vi "TypeDescriptor_GetDefault.vi"(11 "type descriptor":i16[](array[numeric])) -> (0 "error out":errorcluster, 2 "Default":variant, 3 "type descriptor dup":i16[](array[numeric]))   [LabVIEW 2013, in "OpenDescriptor.lvlib"]
uses:
  OpenDescriptor.lvlib
  <vilib>/Utility/error.llb/Error Cluster From Error Code.vi
  <vilib>/ErrorRing/Error Ring.xnode
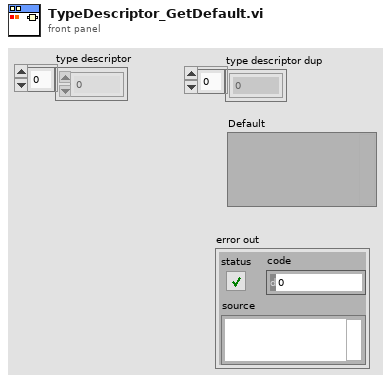
[diagram p1: front panel]
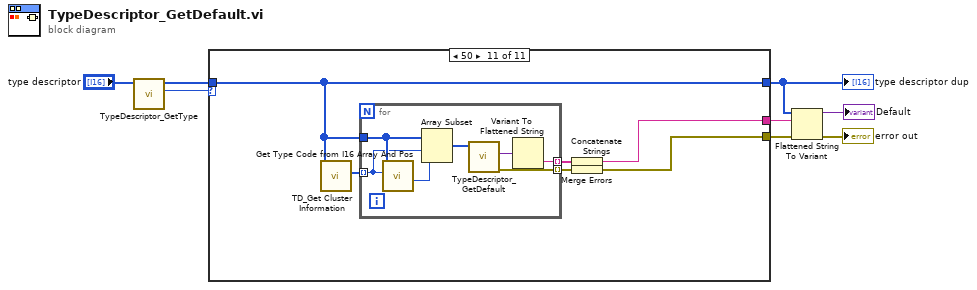
[diagram p0: block diagram]
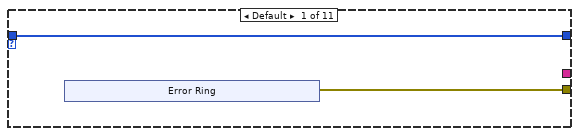
[diagram p2: hidden frame]
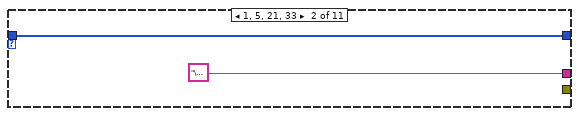
[diagram p3: hidden frame]
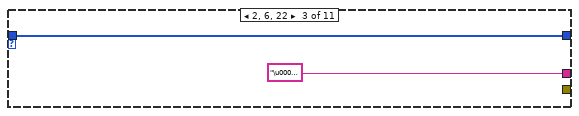
[diagram p4: hidden frame]
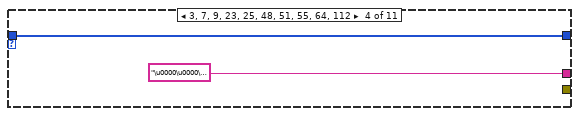
[diagram p5: hidden frame]
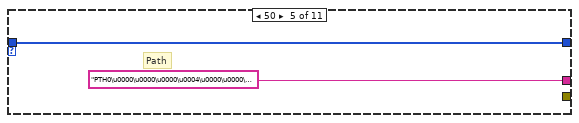
[diagram p6: hidden frame]
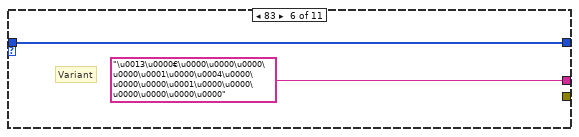
[diagram p7: hidden frame]
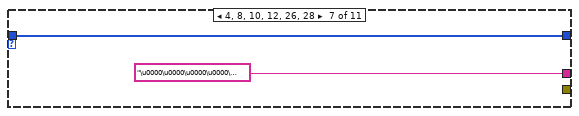
[diagram p8: hidden frame]
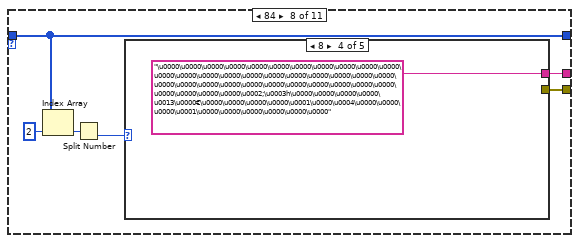
[diagram p9: hidden frame]
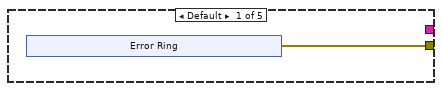
[diagram p10: hidden frame]
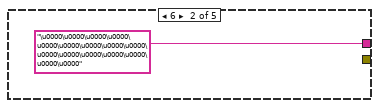
[diagram p11: hidden frame]
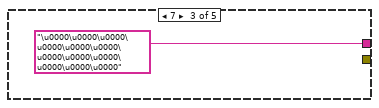
[diagram p12: hidden frame]
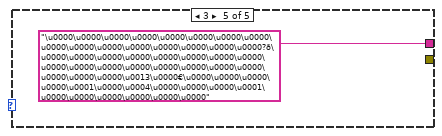
[diagram p13: hidden frame]
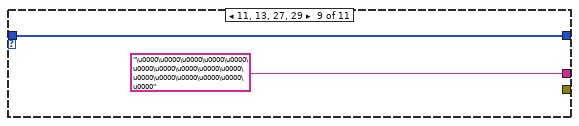
[diagram p14: hidden frame]
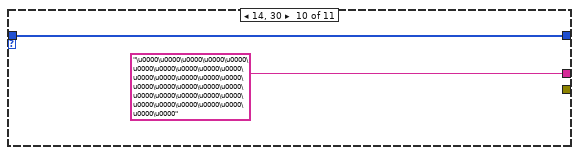
[diagram p15: hidden frame]
diagram:
  n1 = call "TypeDescriptor_GetType.vi"("type descriptor"="type descriptor") -> ("Type"=w7:u8, "type descriptor dup"=w6:i16[])  [unwired: 9 in]
  n2 = case shown="50" w7 {
    tunnel: w6 -> [w10 w17 w19 w20 w23 w25 w27 w30 w45 w47 w51]
    tunnel: [w10 w17 w19 w20 w23 w25 w27 w30 w45 w47 w51] -> w4
    tunnel: [_ "\u0000" ("string") "\u0000\u0000" ("string") "\u0000\u0000\u0000\u0000" ("string") "PTH0\u0000\u0000\u0000\u0004\u0000\u0000\u0000\u0000" ("string") "\u0013\u0000€\u0000\u0000\u0000\u0000\u0001\u0000\u0004\u0000\u0000\u0000\u0001\u0000\u0000\u0000\u0000\u0000\u0000" ("string") "\u0000\u0000\u0000\u0000\u0000\u0000\u0000\u0000" ("string") w33 "\u0000\u0000\u0000\u0000\u0000\u0000\u0000\u0000\u0000\u0000\u0000\u0000\u0000\u0000\u0000\u0000" ("string") "\u0000\u0000\u0000\u0000\u0000\u0000\u0000\u0000\u0000\u0000\u0000\u0000\u0000\u0000\u0000\u0000\u0000\u0000\u0000\u0000\u0000\u0000\u0000\u0000\u0000\u0000\u0000\u0000\u0000\u0000\u0000\u0000" ("string") w50] -> w3
    tunnel: [w9 _ _ _ _ _ _ w28 _ _ w48] -> w1
    frame Default {
      n3 = xnode "Error Ring"() -> ("error out"=w9:errorcluster)
    }
    frame 1, 5, 21, 33 {
    }
    frame 2, 6, 22 {
    }
    frame 3, 7, 9, 23, 25, 48, 51, 55, 64, 112 {
    }
    frame 50 {
      # "Path"
    }
    frame 83 {
      # "Variant"
    }
    frame 4, 8, 10, 12, 26, 28 {
    }
    frame 84 {
      n4 = Index Array(array=w30, index=2) -> (element=w31:i16)
      n5 = Split Number(x=w31) -> (lo(x)=w29:u8)  [unwired: 1 out]
      n6 = case shown="8" w29 {
        tunnel: [_ "\u0000\u0000\u0000\u0000\u0000\u0000\u0000\u0000\u0000\u0000\u0000\u0000\u0000\u0000\u0000\u0000" ("string") "\u0000\u0000\u0000\u0000\u0000\u0000\u0000\u0000\u0000\u0000\u0000\u0000" ("string") "\u0000\u0000\u0000\u0000\u0000\u0000\u0000\u0000\u0000\u0000\u0000\u0000\u0000\u0000\u0000\u0000\u0000\u0000\u0000\u0000\u0000\u0000\u0000\u0000\u0000\u0000\u0000\u0000\u0000\u0000\u0000\u0000\u0000\u0000\u0000\u0000\u0000\u0002;\u0003h\u0000\u0000\u0000\u0000\u0013\u0000€\u0000\u0000\u0000\u0000\u0001\u0000\u0004\u0000\u0000\u0000\u0001\u0000\u0000\u0000\u0000\u0000\u0000" ("string") "\u0000\u0000\u0000\u0000\u0000\u0000\u0000\u0000\u0000\u0000\u0000\u0000\u0000\u0000\u0000\u0000?ð\u0000\u0000\u0000\u0000\u0000\u0000\u0000\u0000\u0000\u0000\u0000\u0000\u0000\u0000\u0000\u0000\u0000\u0000\u0000\u0013\u0000€\u0000\u0000\u0000\u0000\u0001\u0000\u0004\u0000\u0000\u0000\u0001\u0000\u0000\u0000\u0000\u0000\u0000" ("string")] -> w33
        tunnel: [w34 _ _ _ _] -> w28
        frame Default {
          n7 = xnode "Error Ring"() -> ("error out"=w34:errorcluster)
        }
        frame 6 {
        }
        frame 7 {
        }
        frame 8 {
        }
        frame 3 {
        }
      }
    }
    frame 11, 13, 27, 29 {
    }
    frame 14, 30 {
    }
    frame 80 {
      n8 = call <vilib>:"TD_Get Cluster Information.vi"("Type descriptor"=w51) -> ("Contained TD Offsets"=w52:i32[])  [unwired: 9 in, 1 out]
      n9 = for {
        tunnel: w51 -> [w60]
        tunnel: w52 -> [w58] mode=indexing
        tunnel: [w55] -> w53 mode=indexing
        tunnel: [w54] -> w49 mode=indexing
        n10 = call <vilib>:"Get Type Code from I16 Array And Pos.vi"("Pos in Type Descriptor (0)"=w58, "Type descriptor"=w60) -> ("Size (Words)"=w59:i32)  [unwired: 7 in, 2 out]
        n11 = Array Subset(array=w60, index=w58, length=w59) -> (w57:i16[])
        n12 = call "TypeDescriptor_GetDefault.vi"("type descriptor"=w57) -> ("error out"=w54:errorcluster, "Default"=w56:variant)  [unwired: 8 in, 1 out]
        n13 = Variant To Flattened String(Variant=w56) -> (data string=w55:string)  [unwired: 1 out]
      }
      n14 = Concatenate Strings(w53) -> (w50:string)
      n15 = Merge Errors(w49) -> (w48:errorcluster)
    }
  }
  "type descriptor dup" <- w4
  n16 = Flattened String To Variant(4:w1, 6:w3, 7:w4) -> (0:→"error out":errorcluster, 3:→"Default":variant)
